vi "PathPlanner_Holonomic_Create.vi"(4 "Theta Max Accel":dbl format="%20.4f", 6 "Theta Max Speed":dbl format="%20.4f", 8 "error in":errorcluster, 9 "File Name":string="path1.path", 10 "Theta PID Tuning":T11={"Kp"=0.7, "Ki"=0.0, "Kd"=0.0, "MaximumIntegral"=9.9e+30, "MinimumIntegral"=-9.9e+30}, 11 "XY PID Tuning":T11={"Kp"=5.0, "Ki"=0.0, "Kd"=0.0, "MaximumIntegral"=9.9e+30, "MinimumIntegral"=-9.9e+30}) -> (0 "error out":errorcluster, 3 "outPathPlanner_Holonomic":T1={"HOLONOMIC_DRV_CTRL"={"poseTolerance"={"TRANSLATION"={"X"=0.0, "Y"=0.0}, "ROTATION"={"VALUE"=0.0, "COS"=1.0, "SIN"=0.0}}, "poseError"={"TRANSLATION"={"X"=0.0, "Y"=0.0}, "ROTATION"={"VALUE"=0.0, "COS"=1.0, "SIN"=0.0}}, "Enabled"=TRUE, "PID_xCtrl"={"Kp"=0.0, "Ki"=0.0, "Kd"=0.0, "Period"=0.0, "Max_Integral"=1.0, "Min_Integral"=-1.0, "Max_Input"=0.0, "Min_Input"=0.0, "Continuous"=FALSE, "PositionError"=0.0, "VelocityError"=0.0, "PrevError"=0.0, "TotalError"=0.0, "PositionTolerance"=0.05, "VelocityTolerance"=9.99e+35, "SetPoint"=0.0, "Kf"=0.0, "Prev_Deriv"=0.0, "Prev_Deriv 2"=0.0, "DerivativeFilter"=FALSE, "Min_Output"=-9.99e+35, "Max_Output"=9.9e+35, "Prev_F_P"=0.0, "Prev_F_P_2"=0.0, "AntiWindupActive"=FALSE, "Measurement"=0.0}, "PID_yCtrl"={"Kp"=0.0, "Ki"=0.0, "Kd"=0.0, "Period"=0.0, "Max_Integral"=1.0, "Min_Integral"=-1.0, "Max_Input"=0.0, "Min_Input"=0.0, "Continuous"=FALSE, "PositionError"=0.0, "VelocityError"=0.0, "PrevError"=0.0, "TotalError"=0.0, "PositionTolerance"=0.05, "VelocityTolerance"=9.99e+35, "SetPoint"=0.0, "Kf"=0.0, "Prev_Deriv"=0.0, "Prev_Deriv 2"=0.0, "DerivativeFilter"=FALSE, "Min_Output"=-9.99e+35, "Max_Output"=9.9e+35, "Prev_F_P"=0.0, "Prev_F_P_2"=0.0, "AntiWindupActive"=FALSE, "Measurement"=0.0}, "PROF_PID_thetaCtrl"={"Controller"={"Kp"=0.0, "Ki"=0.0, "Kd"=0.0, "Period"=0.0, "Max_Integral"=1.0, "Min_Integral"=-1.0, "Max_Input"=0.0, "Min_Input"=0.0, "Continuous"=FALSE, "PositionError"=0.0, "VelocityError"=0.0, "PrevError"=0.0, "TotalError"=0.0, "PositionTolerance"=0.05, "VelocityTolerance"=9.99e+35, "SetPoint"=0.0, "Kf"=0.0, "Prev_Deriv"=0.0, "Prev_Deriv 2"=0.0, "DerivativeFilter"=FALSE, "Min_Output"=-9.99e+35, "Max_Output"=9.9e+35, "Prev_F_P"=0.0, "Prev_F_P_2"=0.0, "AntiWindupActive"=FALSE, "Measurement"=0.0}, "Goal"={"Position"=0.0, "Velocity"=0.0}, "Setpoint"={"Position"=0.0, "Velocity"=0.0}, "Constraint"={"MaxVelocity"=0.0, "MaxAcceleration"=0.0}}, "RotationError"={"VALUE"=0.0, "COS"=1.0, "SIN"=0.0}, "FirstRun"=FALSE}, "PathPlannerWayPoints"=[]} {"HOLONOMIC_DRV_CTRL"."RotationError"."SIN" format="%13.4f"; "HOLONOMIC_DRV_CTRL"."RotationError"."COS" format="%13.4f"; "HOLONOMIC_DRV_CTRL"."RotationError"."VALUE" format="%13.4f"; "HOLONOMIC_DRV_CTRL"."PROF_PID_thetaCtrl"."Constraint"."MaxAcceleration" format="%16_6e"; "HOLONOMIC_DRV_CTRL"."PROF_PID_thetaCtrl"."Constraint"."MaxVelocity" format="%16_6e"; "HOLONOMIC_DRV_CTRL"."PROF_PID_thetaCtrl"."Setpoint"."Velocity" format="%16_6e"; "HOLONOMIC_DRV_CTRL"."PROF_PID_thetaCtrl"."Setpoint"."Position" format="%16_6e"; "HOLONOMIC_DRV_CTRL"."PROF_PID_thetaCtrl"."Goal"."Velocity" format="%16_6e"; "HOLONOMIC_DRV_CTRL"."PROF_PID_thetaCtrl"."Goal"."Position" format="%16_6e"; "HOLONOMIC_DRV_CTRL"."PROF_PID_thetaCtrl"."Controller"."Measurement" format="%16_6e"; "HOLONOMIC_DRV_CTRL"."PROF_PID_thetaCtrl"."Controller"."Prev_F_P_2" format="%16_6e"; "HOLONOMIC_DRV_CTRL"."PROF_PID_thetaCtrl"."Controller"."Prev_F_P" format="%16_6e"; "HOLONOMIC_DRV_CTRL"."PROF_PID_thetaCtrl"."Controller"."Max_Output" format="%16_6e"; "HOLONOMIC_DRV_CTRL"."PROF_PID_thetaCtrl"."Controller"."Min_Output" format="%16_6e"; "HOLONOMIC_DRV_CTRL"."PROF_PID_thetaCtrl"."Controller"."Prev_Deriv 2" format="%16_6e"; "HOLONOMIC_DRV_CTRL"."PROF_PID_thetaCtrl"."Controller"."Prev_Deriv" format="%16_6e"; "HOLONOMIC_DRV_CTRL"."PROF_PID_thetaCtrl"."Controller"."Kf" format="%16_6e"; "HOLONOMIC_DRV_CTRL"."PROF_PID_thetaCtrl"."Controller"."SetPoint" format="%16_6e"; "HOLONOMIC_DRV_CTRL"."PROF_PID_thetaCtrl"."Controller"."VelocityTolerance" format="%16_6e"; "HOLONOMIC_DRV_CTRL"."PROF_PID_thetaCtrl"."Controller"."PositionTolerance" format="%16_6e"; "HOLONOMIC_DRV_CTRL"."PROF_PID_thetaCtrl"."Controller"."TotalError" format="%16_6e"; "HOLONOMIC_DRV_CTRL"."PROF_PID_thetaCtrl"."Controller"."PrevError" format="%16_6e"; "HOLONOMIC_DRV_CTRL"."PROF_PID_thetaCtrl"."Controller"."VelocityError" format="%16_6e"; "HOLONOMIC_DRV_CTRL"."PROF_PID_thetaCtrl"."Controller"."PositionError" format="%16_6e"; "HOLONOMIC_DRV_CTRL"."PROF_PID_thetaCtrl"."Controller"."Min_Input" format="%16_6e"; "HOLONOMIC_DRV_CTRL"."PROF_PID_thetaCtrl"."Controller"."Max_Input" format="%16_6e"; "HOLONOMIC_DRV_CTRL"."PROF_PID_thetaCtrl"."Controller"."Min_Integral" format="%16_6e"; "HOLONOMIC_DRV_CTRL"."PROF_PID_thetaCtrl"."Controller"."Max_Integral" format="%16_6e"; "HOLONOMIC_DRV_CTRL"."PROF_PID_thetaCtrl"."Controller"."Period" format="%16_6e"; "HOLONOMIC_DRV_CTRL"."PROF_PID_thetaCtrl"."Controller"."Kd" format="%16_6e"; "HOLONOMIC_DRV_CTRL"."PROF_PID_thetaCtrl"."Controller"."Ki" format="%16_6e"; "HOLONOMIC_DRV_CTRL"."PROF_PID_thetaCtrl"."Controller"."Kp" format="%16_6e"; "HOLONOMIC_DRV_CTRL"."PID_yCtrl"."Measurement" format="%16_6e"; "HOLONOMIC_DRV_CTRL"."PID_yCtrl"."Prev_F_P_2" format="%16_6e"; "HOLONOMIC_DRV_CTRL"."PID_yCtrl"."Prev_F_P" format="%16_6e"; "HOLONOMIC_DRV_CTRL"."PID_yCtrl"."Max_Output" format="%16_6e"; "HOLONOMIC_DRV_CTRL"."PID_yCtrl"."Min_Output" format="%16_6e"; "HOLONOMIC_DRV_CTRL"."PID_yCtrl"."Prev_Deriv 2" format="%16_6e"; "HOLONOMIC_DRV_CTRL"."PID_yCtrl"."Prev_Deriv" format="%16_6e"; "HOLONOMIC_DRV_CTRL"."PID_yCtrl"."Kf" format="%16_6e"; "HOLONOMIC_DRV_CTRL"."PID_yCtrl"."SetPoint" format="%16_6e"; "HOLONOMIC_DRV_CTRL"."PID_yCtrl"."VelocityTolerance" format="%16_6e"; "HOLONOMIC_DRV_CTRL"."PID_yCtrl"."PositionTolerance" format="%16_6e"; "HOLONOMIC_DRV_CTRL"."PID_yCtrl"."TotalError" format="%16_6e"; "HOLONOMIC_DRV_CTRL"."PID_yCtrl"."PrevError" format="%16_6e"; "HOLONOMIC_DRV_CTRL"."PID_yCtrl"."VelocityError" format="%16_6e"; "HOLONOMIC_DRV_CTRL"."PID_yCtrl"."PositionError" format="%16_6e"; "HOLONOMIC_DRV_CTRL"."PID_yCtrl"."Min_Input" format="%16_6e"; "HOLONOMIC_DRV_CTRL"."PID_yCtrl"."Max_Input" format="%16_6e"; "HOLONOMIC_DRV_CTRL"."PID_yCtrl"."Min_Integral" format="%16_6e"; "HOLONOMIC_DRV_CTRL"."PID_yCtrl"."Max_Integral" format="%16_6e"; "HOLONOMIC_DRV_CTRL"."PID_yCtrl"."Period" format="%16_6e"; "HOLONOMIC_DRV_CTRL"."PID_yCtrl"."Kd" format="%16_6e"; "HOLONOMIC_DRV_CTRL"."PID_yCtrl"."Ki" format="%16_6e"; "HOLONOMIC_DRV_CTRL"."PID_yCtrl"."Kp" format="%16_6e"; "HOLONOMIC_DRV_CTRL"."PID_xCtrl"."Measurement" format="%16_6e"; "HOLONOMIC_DRV_CTRL"."PID_xCtrl"."Prev_F_P_2" format="%16_6e"; "HOLONOMIC_DRV_CTRL"."PID_xCtrl"."Prev_F_P" format="%16_6e"; "HOLONOMIC_DRV_CTRL"."PID_xCtrl"."Max_Output" format="%16_6e"; "HOLONOMIC_DRV_CTRL"."PID_xCtrl"."Min_Output" format="%16_6e"; "HOLONOMIC_DRV_CTRL"."PID_xCtrl"."Prev_Deriv 2" format="%16_6e"; "HOLONOMIC_DRV_CTRL"."PID_xCtrl"."Prev_Deriv" format="%16_6e"; "HOLONOMIC_DRV_CTRL"."PID_xCtrl"."Kf" format="%16_6e"; "HOLONOMIC_DRV_CTRL"."PID_xCtrl"."SetPoint" format="%16_6e"; "HOLONOMIC_DRV_CTRL"."PID_xCtrl"."VelocityTolerance" format="%16_6e"; "HOLONOMIC_DRV_CTRL"."PID_xCtrl"."PositionTolerance" format="%16_6e"; "HOLONOMIC_DRV_CTRL"."PID_xCtrl"."TotalError" format="%16_6e"; "HOLONOMIC_DRV_CTRL"."PID_xCtrl"."PrevError" format="%16_6e"; "HOLONOMIC_DRV_CTRL"."PID_xCtrl"."VelocityError" format="%16_6e"; "HOLONOMIC_DRV_CTRL"."PID_xCtrl"."PositionError" format="%16_6e"; "HOLONOMIC_DRV_CTRL"."PID_xCtrl"."Min_Input" format="%16_6e"; "HOLONOMIC_DRV_CTRL"."PID_xCtrl"."Max_Input" format="%16_6e"; "HOLONOMIC_DRV_CTRL"."PID_xCtrl"."Min_Integral" format="%16_6e"; "HOLONOMIC_DRV_CTRL"."PID_xCtrl"."Max_Integral" format="%16_6e"; "HOLONOMIC_DRV_CTRL"."PID_xCtrl"."Period" format="%16_6e"; "HOLONOMIC_DRV_CTRL"."PID_xCtrl"."Kd" format="%16_6e"; "HOLONOMIC_DRV_CTRL"."PID_xCtrl"."Ki" format="%16_6e"; "HOLONOMIC_DRV_CTRL"."PID_xCtrl"."Kp" format="%16_6e"; "HOLONOMIC_DRV_CTRL"."poseError"."ROTATION"."SIN" format="%13.4f"; "HOLONOMIC_DRV_CTRL"."poseError"."ROTATION"."COS" format="%13.4f"; "HOLONOMIC_DRV_CTRL"."poseError"."ROTATION"."VALUE" format="%13.4f"; "HOLONOMIC_DRV_CTRL"."poseError"."TRANSLATION"."Y" format="%14.3f"; "HOLONOMIC_DRV_CTRL"."poseError"."TRANSLATION"."X" format="%14.3f"; "HOLONOMIC_DRV_CTRL"."poseTolerance"."ROTATION"."SIN" format="%13.4f"; "HOLONOMIC_DRV_CTRL"."poseTolerance"."ROTATION"."COS" format="%13.4f"; "HOLONOMIC_DRV_CTRL"."poseTolerance"."ROTATION"."VALUE" format="%13.4f"; "HOLONOMIC_DRV_CTRL"."poseTolerance"."TRANSLATION"."Y" format="%14.3f"; "HOLONOMIC_DRV_CTRL"."poseTolerance"."TRANSLATION"."X" format="%14.3f"; "PathPlannerWayPoints"."HolonomicRotation"."SIN" format="%13.4f"; "PathPlannerWayPoints"."HolonomicRotation"."COS" format="%13.4f"; "PathPlannerWayPoints"."HolonomicRotation"."VALUE" format="%13.4f"; "PathPlannerWayPoints"."NextControl"."Y" format="%14.3f"; "PathPlannerWayPoints"."NextControl"."X" format="%14.3f"; "PathPlannerWayPoints"."PrevControl"."Y" format="%14.3f"; "PathPlannerWayPoints"."PrevControl"."X" format="%14.3f"; "PathPlannerWayPoints"."AnchorPoint"."Y" format="%14.3f"; "PathPlannerWayPoints"."AnchorPoint"."X" format="%14.3f"})   [LabVIEW 2020]
doc: "Loads a <B>PathPlanner</B> trajectory file."
uses:
  <vilib>/Rock Robotics/WPI/ThirdParty/JAS_Junk/TrajLib/PID_TUNING.ctl
  PathPlanner_Holonomic.ctl
  <vilib>/Rock Robotics/WPI/ThirdParty/JAS_Junk/TrajLib/HOLONOMIC_DRV_CTRL.ctl
  <vilib>/Rock Robotics/WPI/ThirdParty/JAS_Junk/TrajLib/POSE2D.ctl
  <vilib>/Rock Robotics/WPI/ThirdParty/JAS_Junk/TrajLib/TRANSLATION2D.ctl
  <vilib>/Rock Robotics/WPI/ThirdParty/JAS_Junk/TrajLib/ROTATION2D.ctl
  <vilib>/Rock Robotics/WPI/ThirdParty/JAS_Junk/TrajLib/PID_CONTROLLER.ctl
  <vilib>/Rock Robotics/WPI/ThirdParty/JAS_Junk/TrajLib/PROFILED_PID_CONTROLLER.ctl
  <vilib>/Rock Robotics/WPI/ThirdParty/JAS_Junk/TrajLib/TRAPEZOID_PROFILE_STATE.ctl
  <vilib>/Rock Robotics/WPI/ThirdParty/JAS_Junk/TrajLib/TRAPEZOID_PROFILE_CONSTRAINT.ctl
  <vilib>/Rock Robotics/WPI/ThirdParty/MJansen/PathPlanner/PathPlannerWaypoint.ctl
  <vilib>/Rock Robotics/WPI/ThirdParty/JAS_Junk/TrajLib/ProfiledPIDController_NewPeriod.vi
  <vilib>/Rock Robotics/WPI/ThirdParty/JAS_Junk/TrajLib/ProfiledPIDController_SetIntegratorRange.vi
  <vilib>/Rock Robotics/WPI/ThirdParty/JAS_Junk/TrajLib/ProfiledPIDController_DisableContInput.vi
  <vilib>/Rock Robotics/WPI/ThirdParty/JAS_Junk/TrajLib/ProfiledPIDController_EnableContInput.vi
  <vilib>/Rock Robotics/WPI/ThirdParty/JAS_Junk/TrajLib/TrapProfConstraint_New.vi
  <vilib>/Rock Robotics/WPI/ThirdParty/JAS_Junk/TrajLib/PIDController_NewPeriod.vi
  <vilib>/Rock Robotics/WPI/ThirdParty/JAS_Junk/TrajLib/PIDController_SetIntegratorRange.vi
  <vilib>/Rock Robotics/WPI/ThirdParty/JAS_Junk/TrajLib/PIDController_Reset.vi
  <vilib>/Rock Robotics/WPI/ThirdParty/JAS_Junk/TrajLib/TrapProfState_New.vi
  <vilib>/Rock Robotics/SystemInterfaces/NetworkCommunication/NetComm_UsageReport_report.vi
  <vilib>/Rock Robotics/WPI/ThirdParty/JAS_Junk/TrajLib/PIDController_DisableContinousInput.vi
  <vilib>/Rock Robotics/WPI/ThirdParty/JAS_Junk/TrajLib/PIDController_EnableContinousInput.vi
  <vilib>/Rock Robotics/WPI/ThirdParty/JAS_Junk/TrajLib/Util_LibraryGlobals.vi
  <vilib>/Rock Robotics/WPI/ThirdParty/JAS_Junk/TrajLib/Trajectory_Library.lvlib
  <vilib>/Rock Robotics/WPI/ThirdParty/MJansen/PathPlanner/PathPlanner.lvlib
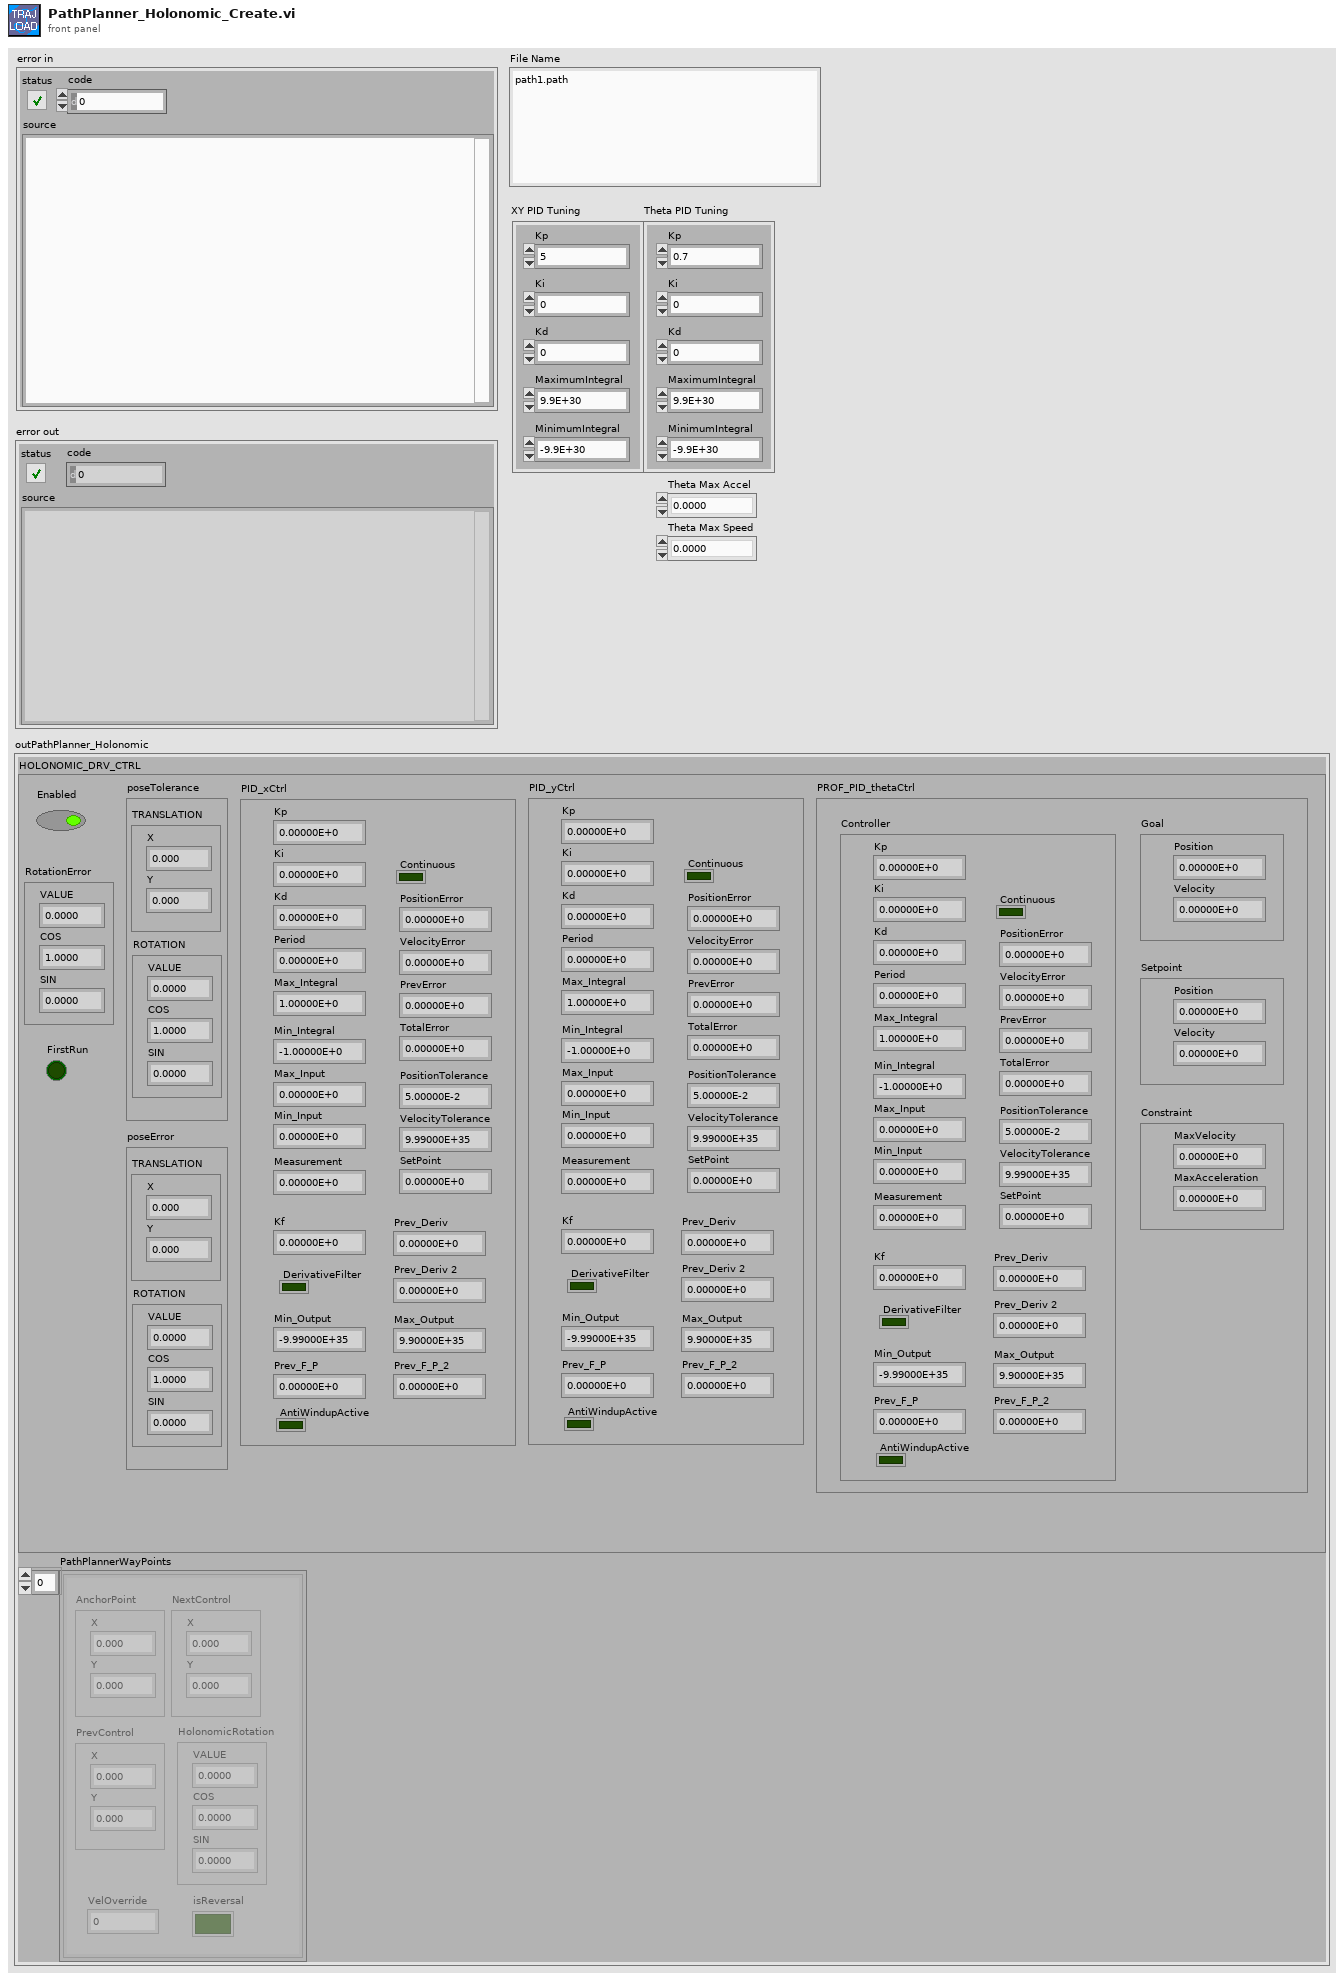
[diagram p1: front panel]
types:
  T1 = typedef "PathPlanner_Holonomic.ctl" = cluster{"HOLONOMIC_DRV_CTRL":T2, "PathPlannerWayPoints":T10[]}
  T2 = typedef "Trajectory_Library.lvlib/HOLONOMIC_DRV_CTRL.ctl" = cluster{"poseTolerance":T3, "poseError":T3, "Enabled":bool, "PID_xCtrl":T6, "PID_yCtrl":T6, "PROF_PID_thetaCtrl":T7, "RotationError":T5, "FirstRun":bool}
  T3 = typedef "Trajectory_Library.lvlib/POSE2D.ctl" = cluster{"TRANSLATION":T4, "ROTATION":T5}
  T4 = typedef "Trajectory_Library.lvlib/TRANSLATION2D.ctl" = cluster{"X":dbl, "Y":dbl}
  T5 = typedef "Trajectory_Library.lvlib/ROTATION2D.ctl" = cluster{"VALUE":dbl, "COS":dbl, "SIN":dbl}
  T6 = typedef "Trajectory_Library.lvlib/PID_CONTROLLER.ctl" = cluster{"Kp":dbl, "Ki":dbl, "Kd":dbl, "Period":dbl, "Max_Integral":dbl, "Min_Integral":dbl, "Max_Input":dbl, "Min_Input":dbl, "Continuous":bool, "PositionError":dbl, "VelocityError":dbl, "PrevError":dbl, "TotalError":dbl, "PositionTolerance":dbl, "VelocityTolerance":dbl, "SetPoint":dbl, "Kf":dbl, "Prev_Deriv":dbl, "Prev_Deriv 2":dbl, "DerivativeFilter":bool, "Min_Output":dbl, "Max_Output":dbl, "Prev_F_P":dbl, "Prev_F_P_2":dbl, "AntiWindupActive":bool, "Measurement":dbl}
  T7 = typedef "Trajectory_Library.lvlib/PROFILED_PID_CONTROLLER.ctl" = cluster{"Controller":T6, "Goal":T8, "Setpoint":T8, "Constraint":T9}
  T8 = typedef "Trajectory_Library.lvlib/TRAPEZOID_PROFILE_STATE.ctl" = cluster{"Position":dbl, "Velocity":dbl}
  T9 = typedef "Trajectory_Library.lvlib/TRAPEZOID_PROFILE_CONSTRAINT.ctl" = cluster{"MaxVelocity":dbl, "MaxAcceleration":dbl}
  T10 = typedef "PathPlanner.lvlib/PathPlannerWaypoint.ctl" = cluster{"AnchorPoint":T4, "PrevControl":T4, "NextControl":T4, "HolonomicRotation":T5, "VelOverride":dbl, "isReversal":bool}
  T11 = typedef "Trajectory_Library.lvlib/PID_TUNING.ctl" = cluster{"Kp":dbl, "Ki":dbl, "Kd":dbl, "MaximumIntegral":dbl, "MinimumIntegral":dbl}
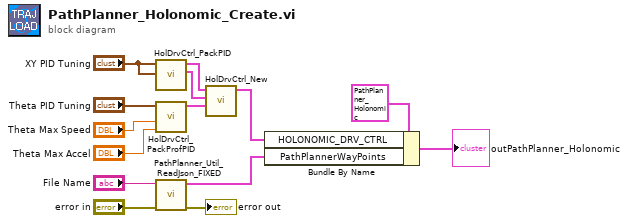
[diagram p0: block diagram]
diagram:
  n1 = call <vilib>:"HolDrvCtrl_PackPID.vi"("Y PID Tuning"="XY PID Tuning", "X PID Tuning"="XY PID Tuning") -> ("Y PID CONTROLLER"=w10:T6, "X PID_CONTROLLER"=w11:T6)  [unwired: 8 in]
  n2 = call <vilib>:"HolDrvCtrl_PackProfPID.vi"("Max Accel"="Theta Max Accel", "Max Speed"="Theta Max Speed", "Theta PID Tuning"="Theta PID Tuning") -> ("Theta PID CONTROLLER"=w13:T7)  [unwired: 8 in]
  n3 = call "PathPlanner_Util_ReadJson_FIXED.vi"("error in (no error)"="error in", "FileName"="File Name") -> ("error out"=→"error out":errorcluster, "PathPlannerWayPoints"=w3:T10[])  [unwired: 7 in, 1 out]
  n4 = call <vilib>:"HolDrvCtrl_New.vi"("thetaProfiledPID_CTRL"=w13, "yPID_CTRL"=w10, "xPID_CTRL"=w11) -> ("outHOLONOMIC_DRV_CTRL"=w4:T2)  [unwired: 8 in]
  n5 = Bundle By Name(cluster=T1 {"HOLONOMIC_DRV_CTRL"={"poseTolerance"={"TRANSLATION"={"X"=0.0, "Y"=0.0}, "ROTATION"={"VALUE"=0.0, "COS"=1.0, "SIN"=0.0}}, "poseError"={"TRANSLATION"={"X"=0.0, "Y"=0.0}, "ROTATION"={"VALUE"=0.0, "COS"=1.0, "SIN"=0.0}}, "Enabled"=TRUE, "PID_xCtrl"={"Kp"=0.0, "Ki"=0.0, "Kd"=0.0, "Period"=0.0, "Max_Integral"=1.0, "Min_Integral"=-1.0, "Max_Input"=0.0, "Min_Input"=0.0, "Continuous"=FALSE, "PositionError"=0.0, "VelocityError"=0.0, "PrevError"=0.0, "TotalError"=0.0, "PositionTolerance"=0.05, "VelocityTolerance"=9.99e+35, "SetPoint"=0.0, "Kf"=0.0, "Prev_Deriv"=0.0, "Prev_Deriv 2"=0.0, "DerivativeFilter"=FALSE, "Min_Output"=-9.99e+35, "Max_Output"=9.9e+35, "Prev_F_P"=0.0, "Prev_F_P_2"=0.0, "AntiWindupActive"=FALSE, "Measurement"=0.0}, "PID_yCtrl"={"Kp"=0.0, "Ki"=0.0, "Kd"=0.0, "Period"=0.0, "Max_Integral"=1.0, "Min_Integral"=-1.0, "Max_Input"=0.0, "Min_Input"=0.0, "Continuous"=FALSE, "PositionError"=0.0, "VelocityError"=0.0, "PrevError"=0.0, "TotalError"=0.0, "PositionTolerance"=0.05, "VelocityTolerance"=9.99e+35, "SetPoint"=0.0, "Kf"=0.0, "Prev_Deriv"=0.0, "Prev_Deriv 2"=0.0, "DerivativeFilter"=FALSE, "Min_Output"=-9.99e+35, "Max_Output"=9.9e+35, "Prev_F_P"=0.0, "Prev_F_P_2"=0.0, "AntiWindupActive"=FALSE, "Measurement"=0.0}, "PROF_PID_thetaCtrl"={"Controller"={"Kp"=0.0, "Ki"=0.0, "Kd"=0.0, "Period"=0.0, "Max_Integral"=1.0, "Min_Integral"=-1.0, "Max_Input"=0.0, "Min_Input"=0.0, "Continuous"=FALSE, "PositionError"=0.0, "VelocityError"=0.0, "PrevError"=0.0, "TotalError"=0.0, "PositionTolerance"=0.05, "VelocityTolerance"=9.99e+35, "SetPoint"=0.0, "Kf"=0.0, "Prev_Deriv"=0.0, "Prev_Deriv 2"=0.0, "DerivativeFilter"=FALSE, "Min_Output"=-9.99e+35, "Max_Output"=9.9e+35, "Prev_F_P"=0.0, "Prev_F_P_2"=0.0, "AntiWindupActive"=FALSE, "Measurement"=0.0}, "Goal"={"Position"=0.0, "Velocity"=0.0}, "Setpoint"={"Position"=0.0, "Velocity"=0.0}, "Constraint"={"MaxVelocity"=0.0, "MaxAcceleration"=0.0}}, "RotationError"={"VALUE"=0.0, "COS"=1.0, "SIN"=0.0}, "FirstRun"=FALSE}, "PathPlannerWayPoints"=[]}, "HOLONOMIC_DRV_CTRL"=w4, "PathPlannerWayPoints"=w3) -> (→"outPathPlanner_Holonomic":T1)
